vi "WorkorderHandler_LoadFile.vi"(8 "error in (no error)":errorcluster, 11 "reference":T1) -> (0 "error out":errorcluster, 3 "duplicate reference":T1)   [LabVIEW 2011]
uses:
  DataStructures/WorkorderHandler_ObjectReference.ctl
  Strict Type Controls/Settings Operation.ctl
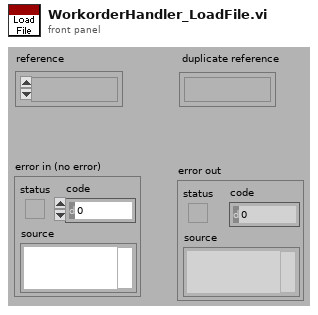
[diagram p1: front panel]
types:
  T1 = typedef "WorkorderHandler_ObjectReference.ctl" = refnum<k1>
  T2 = typedef "WorkorderHandler_ObjectData.ctl" = cluster{"Table":string[][], "Script":string, "Order":string, "No":string, "Time":dbl}
  T3 = typedef "Settings Operation.ctl" = enum8{"Get Value", "Set Value", "Read File", "Write File", "Write Stored Value"}
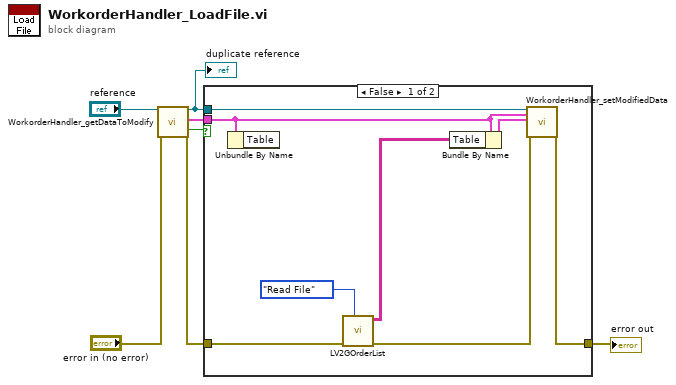
[diagram p0: block diagram]
diagram:
  n1 = call "WorkorderHandler_getDataToModify.vi"("reference"="reference", "error in (no error)"="error in (no error)") -> ("duplicate reference"=w3:T1, "data"=w6:T2, "timed out?"=w1:bool, "error out"=w2:errorcluster)  [unwired: 1 in, 13 out]
  "duplicate reference" <- w3
  n2 = case shown="False" w1 {
    tunnel: [w14 w16] -> w7
    tunnel: w6 -> [w12 _]
    tunnel: w3 -> [w15 _]
    tunnel: w2 -> [w11 w16]
    frame False {
      n3 = Unbundle By Name(w12) -> ()  [unwired: 1 out]
      n4 = call "LV2GOrderList.vi"("Operation"=Settings_Operation."Read File", "error in (no error)"=w11) -> ("error out"=w10:errorcluster, "Orders out"=w8:string[][])  [unwired: 1 in, 7 out]
      n5 = Bundle By Name(cluster=w12, "Table"=w8) -> (w13:T2)
      n6 = call "WorkorderHandler_setModifiedData.vi"("reference"=w15, "data (unmodified)"=w12, "data"=w13, "error in (no error)"=w10) -> ("error out"=w14:errorcluster)  [unwired: 15 out]
    }
    frame True {
      # "Error or Timed Out"
    }
  }
  "error out" <- w7
